vi "BMU诊断标定.vi"(5 "timeout":u32, 6 "Socket":dbl, 7 "通用配置?":bool, 8 "CAN端口":u16(ring), 9 "设备索引号":u16(ring), 10 "CAN卡类型":u32(ring)=21, 11 "从板号":u8=1) -> (3 "成功?":bool)   [LabVIEW 2013] (continued)
                              n874 = local write "正级继电器 8"(w1437) -> ()
                            }
                            frame 85, 170 {
                              n875 = local write "继电器超时处理"(TRUE ("继电器超时处理")) -> ()
                            }
                          }
                        }
                        frame 2 {
                          n876 = Index Array(array=w1453) -> (element #1=w1452:u8, element #2=w1451:u8, element #3=w1450:u8)  [unwired: 3 in]
                          n877 = Join Numbers(hi=w1451, lo=w1450) -> ((hi.lo)=w1449:u16)
                          n878 = case shown="2" w1452 {
                            tunnel: w1453 -> [_ _ _]
                            tunnel: w1449 -> [_ w1457 w1471]
                            tunnel: w1448 -> [_ w1456 _]
                            frame 0, Default {
                              n879 = local write "继电器超时处理"(FALSE ("继电器超时处理")) -> ()
                            }
                            frame 1 {
                              n880 = Equal To 0?(x=w1457) -> (x = 0?=w1455:bool)
                              n881 = case shown="假" w1455 {
                                tunnel: w1457 -> [w1463 _]
                                tunnel: [w1461 "DO控制操作成功!\nDO控制操作成功!\nDO控制操作成功!"] -> _
                                tunnel: w1456 -> [w1460 _]
                                frame False {
                                n882 = case shown="\"主板\", 默认" w1460 {
                                frame "主板", Default {
                                n883 = local read "DO1"() -> (w1466:bool)
                                n884 = Not(x=w1466) -> (.not. x?=w1465:bool)
                                n885 = local write "DO1"(w1465) -> ()
                                }
                                frame "从板" {
                                n886 = local read "DO1 2"() -> (w1468:bool)
                                n887 = Not(x=w1468) -> (.not. x?=w1467:bool)
                                n888 = local write "DO1 2"(w1467) -> ()
                                }
                                }
                                n889 = Number To Hexadecimal String(2:w1463) -> (0:w1462:string)  [unwired: 1 out]
                                n890 = Concatenate Strings("DO控制操作失败,0x" ("消息"), w1462) -> (w1461:string)
                                }
                                frame True {
                                }
                              }
                              n891 = case shown="\"从板\"" w1456 {
                                tunnel: w1455 -> [w1458 w1459]
                                frame "主板", Default {
                                n892 = local write "正级继电器 9"(w1458) -> ()
                                }
                                frame "从板" {
                                n893 = local write "正级继电器 11"(w1459) -> ()
                                }
                              }
                            }
                            frame 2 {
                              n894 = Equal To 0?(x=w1471) -> (x = 0?=w1470:bool)
                              n895 = case shown="假" w1470 {
                                tunnel: w1471 -> [w1476 _]
                                tunnel: [w1474 "DO控制操作成功!\nDO控制操作成功!\nDO控制操作成功!"] -> _
                                frame False {
                                n896 = Number To Hexadecimal String(2:w1476) -> (0:w1475:string)  [unwired: 1 out]
                                n897 = local read "DO2"() -> (w1473:bool)
                                n898 = Not(x=w1473) -> (.not. x?=w1472:bool)
                                n899 = Concatenate Strings("DO控制操作失败,0x" ("消息"), w1475) -> (w1474:string)
                                n900 = local write "DO2"(w1472) -> ()
                                }
                                frame True {
                                }
                              }
                              n901 = local write "正级继电器 10"(w1470) -> ()
                            }
                          }
                        }
                      }
                      n902 = local write "消除"(FALSE ("消除")) -> ()
                      n903 = global write "EV05全局变量1.vi" "流控帧 2"(FALSE ("流控帧 2")) -> ()
                      n904 = local write "控制1"(FALSE ("控制1")) -> ()
                      "继电器超时处理" <- TRUE ("控制1")
                    }
                  }
                }
                frame "高压板校正" {
                  n905 = local read "命令序号"() -> (w1483:u8)
                  n906 = call "多帧接收机制(EV05).vi"("can卡类型"=w1490, "设备索引号"=w1489, "CAN端口"=w1488, "VCI_Receive"=w1487, "命令"=w1485, "板号"=w1486, "命令序号"=w1483) -> ("错误信号"=w1479:bool, "错误代码"=w1492:i32, "输出数组"=w1484:u8[], "读错误代码"=w1482:u8[], "结束信号"=w1491:bool)  [unwired: 3 in, 5 out]
                  n907 = local read "控制1"() -> (w1480:bool)
                  n908 = And(x=w1480, y=w1491) -> (x .and. y?=w1481:bool)
                  n909 = case shown="真" w1481 {
                    tunnel: w1493 -> [_ w1497]
                    tunnel: w1492 -> [_ _]
                    tunnel: w1484 -> [_ w1495]
                    tunnel: w1483 -> [_ w1496]
                    tunnel: w1482 -> [_ w1498]
                    tunnel: w1479 -> [_ w1499]
                    frame False {
                    }
                    frame True {
                      n910 = case shown="假" w1499 {
                        tunnel: w1498 -> [_ w1709]
                        tunnel: w1497 -> [_ _]
                        tunnel: w1496 -> [w1504 _]
                        tunnel: w1495 -> [w1503 _]
                        frame False {
                          n911 = case shown="2" w1504 {
                            tunnel: w1503 -> [_ w1509 w1543 w1573 w1600 w1627 w1654 w1681]
                            frame 0, Default {
                            }
                            frame 1 {
                              n912 = for {
                                N: 10 -> [_]
                                tunnel: w1509 -> [w1526]
                                shift-right: [w1513] -> w1507
                                shift-left: string[] [] -> [w1515]
                                i -> [w1512]
                                w1520 = 8 ("索引")
                                w1524 = 2 ("y")
                                n913 = Multiply(x=w1512, y=w1524) -> (x*y=w1525:i32)
                                n914 = Array Subset(array=w1526, index=w1525, length=w1524) -> (w1523:u8[])
                                n915 = Index Array(array=w1523) -> (element #1=w1522:u8, element #2=w1521:u8)  [unwired: 2 in]
                                n916 = call "二进制解析-8.6.vi"("索引"=w1520, "数值"=w1522) -> ("低位子数组"=w1519:i32[])  [unwired: 1 in, 2 out]
                                n917 = call "二进制解析-8.6.vi"("索引"=w1520, "数值"=w1521) -> ("低位子数组"=w1518:i32[])  [unwired: 1 in, 2 out]
                                n918 = Insert Into Array(array=w1519, new element=w1518) -> (w1517:i32[])  [unwired: 1 in]
                                n919 = case shown="2" w1512 {
                                tunnel: [6 15 9 4 2 0 2] -> w1511
                                frame 0, Default {
                                }
                                frame 1 {
                                }
                                frame 2 {
                                }
                                frame 3..5 {
                                }
                                frame 8, 9 {
                                }
                                frame 7 {
                                }
                                frame 6 {
                                }
                                }
                                n920 = Reverse 1D Array(array=w1517) -> (reversed array=w1516:i32[])
                                n921 = for {
                                N: w1511 -> [_]
                                tunnel: w1516 -> [w1538] mode=indexing
                                tunnel: [w1534] -> w1514 mode=indexing
                                n922 = Equal To 0?(x=w1538) -> (x = 0?=w1537:bool)
                                n923 = Select(t="无", s=w1537, f="故障") -> (s? t:f=w1534:string)
                                }
                                n924 = Insert Into Array(array=w1515, new element=w1514) -> (w1513:string[])  [unwired: 1 in]
                              }
                              n925 = call "详细故障分解.vi"("名称"=string[] ["上电自检异常(CellV)", "通讯异常(CellV)", "不更新(CellV)", "未校准(CellV)", "保留", "采样线路断路(CellV)", "18b20上电自检异常(T) ", "18b20通讯异常(T)", "18b20传感器丢失(T)", "18b20传感器无号(T)", "18b20温度异常跳变(T)", "18b20信号线对电源短路(T)", "18b20信号线对地短路(T)", "18b20 CRC校验异常(T)", "NTC上电自检异常(T)", "NTC通讯异常(T)", "NTC传感器丢失(T)", "NTC温度异常跳变(T)", "NTC信号线断路(T)", "NTC信号线对电源短(T)", "NTC信号线对地短路(T)", "上电自检异常(Curr)", "参数异常(Curr)", "不更新(Curr)", "未校准(Curr)", "采样线断开(Curr)", "电流零漂异常(Curr)", "传感器反接(Curr)", "读取实时电流故障(Curr)", "平均电流故障(Curr)", "自检异常(iso)", "前端检测电阻损坏(iso)", "不更新(iso)", "未校准(iso)", "上电自检异常(Sumv_in)", "通讯异常(Sumv_in)", "不更新(Sumv_in)", "未校准(Sumv_in)", "上电自检异常(Sumv_out)", "通讯异常(Sumv_out)", "不更新(Sumv_out)", "未校准(Sumv_out)", "系统时钟自检异常(Clock)", "系统时钟未校准(Clock)", "充电均衡模块不能开启", "充电均衡模块不能关闭", "放电均衡模块不能开启", "放电均衡模块不能关闭"], "故障输入口"=w1507) -> ("输出数组"=w1505:string[][])  [unwired: 1 in, 2 out]
                              n926 = local write "电池故障"(w1505) -> ()
                            }
                            frame 2 {
                              n927 = for {
                                N: 5 -> [_]
                                tunnel: w1543 -> [w1560]
                                shift-right: [w1547] -> w1541
                                shift-left: string[] [] -> [w1549]
                                i -> [w1545]
                                w1554 = 8 ("索引")
                                w1558 = 2 ("y")
                                n928 = Multiply(x=w1545, y=w1558) -> (x*y=w1559:i32)
                                n929 = Array Subset(array=w1560, index=w1559, length=w1558) -> (w1557:u8[])
                                n930 = Index Array(array=w1557) -> (element #1=w1556:u8, element #2=w1555:u8)  [unwired: 2 in]
                                n931 = call "二进制解析-8.6.vi"("索引"=w1554, "数值"=w1556) -> ("低位子数组"=w1553:i32[])  [unwired: 1 in, 2 out]
                                n932 = call "二进制解析-8.6.vi"("索引"=w1554, "数值"=w1555) -> ("低位子数组"=w1552:i32[])  [unwired: 1 in, 2 out]
                                n933 = Insert Into Array(array=w1553, new element=w1552) -> (w1551:i32[])  [unwired: 1 in]
                                n934 = case shown="2" w1545 {
                                tunnel: [4 6 5] -> w1546
                                frame 0, Default {
                                }
                                frame 2 {
                                }
                                frame 4 {
                                }
                                }
                                n935 = Reverse 1D Array(array=w1551) -> (reversed array=w1550:i32[])
                                n936 = for {
                                N: w1546 -> [_]
                                tunnel: w1550 -> [w1568] mode=indexing
                                tunnel: [w1564] -> w1548 mode=indexing
                                n937 = Equal To 0?(x=w1568) -> (x = 0?=w1567:bool)
                                n938 = Select(t="无", s=w1567, f="故障") -> (s? t:f=w1564:string)
                                }
                                n939 = Insert Into Array(array=w1549, new element=w1548) -> (w1547:string[])  [unwired: 1 in]
                              }
                              n940 = call "详细故障分解.vi"("名称"=string[] ["自检异常(ee_cpu)", "存储空间满(ee_cpu)", "数据写入失败(ee_cpu)", "数据读取异常(ee_cpu)", "自检异常(ee_ext)", "存储空间满(ee_ext)", "数据写入失败(ee_ext)", "数据读取异常(ee_ext)", "自检异常(flash_ext)", "故障数据存储空间满(flash_ext)", "历史数据存储空间满(flash_ext)", "数据写入失败(flash_ext)", "数据读取失败(flash_ext)", "数据校验异常(flash_ext)", "自检异常(flash_cpu)", "存储空间满(flash_cpu)", "数据写入失败(flash_cpu)", "数据读取异常(flash_cpu)", "应用程序异常(cpu)", "应用程序下载异常(cpu)", "AD模块异常(cpu)", "RAM异常(cpu)", "CPU异常下电(cpu)"], "故障输入口"=w1541) -> ("输出数组"=w1539:string[][])  [unwired: 1 in, 2 out]
                              n941 = local write "电池故障"(w1539) -> ()
                            }
                            frame 3 {
                              n942 = for {
                                N: 5 -> [_]
                                tunnel: w1573 -> [w1590]
                                shift-right: [w1577] -> w1571
                                shift-left: string[] [] -> [w1579]
                                i -> [w1576]
                                w1584 = 8 ("索引")
                                w1588 = 2 ("y")
                                n943 = Multiply(x=w1576, y=w1588) -> (x*y=w1589:i32)
                                n944 = Array Subset(array=w1590, index=w1589, length=w1588) -> (w1587:u8[])
                                n945 = Index Array(array=w1587) -> (element #1=w1586:u8, element #2=w1585:u8)  [unwired: 2 in]
                                n946 = call "二进制解析-8.6.vi"("索引"=w1584, "数值"=w1586) -> ("低位子数组"=w1583:i32[])  [unwired: 1 in, 2 out]
                                n947 = call "二进制解析-8.6.vi"("索引"=w1584, "数值"=w1585) -> ("低位子数组"=w1582:i32[])  [unwired: 1 in, 2 out]
                                n948 = Insert Into Array(array=w1583, new element=w1582) -> (w1581:i32[])  [unwired: 1 in]
                                n949 = Reverse 1D Array(array=w1581) -> (reversed array=w1580:i32[])
                                n950 = for {
                                N: 6 -> [_]
                                tunnel: w1580 -> [w1595] mode=indexing
                                tunnel: [w1591] -> w1578 mode=indexing
                                n951 = Equal To 0?(x=w1595) -> (x = 0?=w1594:bool)
                                n952 = Select(t="无", s=w1594, f="故障") -> (s? t:f=w1591:string)
                                }
                                n953 = Insert Into Array(array=w1579, new element=w1578) -> (w1577:string[])  [unwired: 1 in]
                              }
                              n954 = call "详细故障分解.vi"("名称"=string[] ["初始化失败(CAN4)", "发送异常(CAN4)", "接收异常(CAN4)", "总线超时(CAN4)", "BUSOFF(CAN4)", "帧格式(CAN4)", "初始化异常(CAN0)", "发送异常(CAN0)", "接收异常(CAN0)", "总线超时(CAN0)", "BUSOFF(CAN0)", "帧格式(CAN0)", "初始化异常(CAN1)", "发送异常(CAN1)", "接收异常(CAN1)", "总线超时(CAN1)", "BUSOFF(CAN1)", "帧格式(CAN1)", "初始化失败(CAN2)", "发送异常(CAN2)", "接收异常(CAN2)", "总线超时(CAN2)", "BUSOFF(CAN2)", "帧格式(CAN2)", "初始化失败(CAN3)", "发送异常(CAN3)", "接收异常(CAN3)", "总线超时(CAN3)", "BUSOFF(CAN3)", "帧格式(CAN3)"], "故障输入口"=w1571) -> ("输出数组"=w1569:string[][])  [unwired: 1 in, 2 out]
                              n955 = local write "电池故障"(w1569) -> ()
                            }
                            frame 4 {
                              n956 = for {
                                N: 1 -> [_]
                                tunnel: w1600 -> [w1617]
                                shift-right: [w1604] -> w1598
                                shift-left: string[] [] -> [w1606]
                                i -> [w1603]
                                w1611 = 8 ("索引")
                                w1615 = 2 ("y")
                                n957 = Multiply(x=w1603, y=w1615) -> (x*y=w1616:i32)
                                n958 = Array Subset(array=w1617, index=w1616, length=w1615) -> (w1614:u8[])
                                n959 = Index Array(array=w1614) -> (element #1=w1613:u8, element #2=w1612:u8)  [unwired: 2 in]
                                n960 = call "二进制解析-8.6.vi"("索引"=w1611, "数值"=w1613) -> ("低位子数组"=w1610:i32[])  [unwired: 1 in, 2 out]
                                n961 = call "二进制解析-8.6.vi"("索引"=w1611, "数值"=w1612) -> ("低位子数组"=w1609:i32[])  [unwired: 1 in, 2 out]
                                n962 = Insert Into Array(array=w1610, new element=w1609) -> (w1608:i32[])  [unwired: 1 in]
                                n963 = Reverse 1D Array(array=w1608) -> (reversed array=w1607:i32[])
                                n964 = for {
                                N: 4 -> [_]
                                tunnel: w1607 -> [w1622] mode=indexing
                                tunnel: [w1618] -> w1605 mode=indexing
                                n965 = Equal To 0?(x=w1622) -> (x = 0?=w1621:bool)
                                n966 = Select(t="无", s=w1621, f="故障") -> (s? t:f=w1618:string)
                                }
                                n967 = Insert Into Array(array=w1606, new element=w1605) -> (w1604:string[])  [unwired: 1 in]
                              }
                              n968 = call "详细故障分解.vi"("名称"=string[] ["通讯协议版本不一致(soft)", "系统不同步(soft)", "软件版本不一致(soft)", "同硬件平台不兼容(soft)"], "故障输入口"=w1598) -> ("输出数组"=w1596:string[][])  [unwired: 1 in, 2 out]
                              n969 = local write "电池故障"(w1596) -> ()
                            }
                            frame 5 {
                              n970 = for {
                                N: 2 -> [_]
                                tunnel: w1627 -> [w1644]
                                shift-right: [w1631] -> w1625
                                shift-left: string[] [] -> [w1633]
                                i -> [w1630]
                                w1638 = 8 ("索引")
                                w1642 = 2 ("y")
                                n971 = Multiply(x=w1630, y=w1642) -> (x*y=w1643:i32)
                                n972 = Array Subset(array=w1644, index=w1643, length=w1642) -> (w1641:u8[])
                                n973 = Index Array(array=w1641) -> (element #1=w1640:u8, element #2=w1639:u8)  [unwired: 2 in]
                                n974 = call "二进制解析-8.6.vi"("索引"=w1638, "数值"=w1640) -> ("低位子数组"=w1637:i32[])  [unwired: 1 in, 2 out]
                                n975 = call "二进制解析-8.6.vi"("索引"=w1638, "数值"=w1639) -> ("低位子数组"=w1636:i32[])  [unwired: 1 in, 2 out]
                                n976 = Insert Into Array(array=w1637, new element=w1636) -> (w1635:i32[])  [unwired: 1 in]
                                n977 = Reverse 1D Array(array=w1635) -> (reversed array=w1634:i32[])
                                n978 = for {
                                N: 4 -> [_]
                                tunnel: w1634 -> [w1649] mode=indexing
                                tunnel: [w1645] -> w1632 mode=indexing
                                n979 = Equal To 0?(x=w1649) -> (x = 0?=w1648:bool)
                                n980 = Select(t="无", s=w1648, f="故障") -> (s? t:f=w1645:string)
                                }
                                n981 = Insert Into Array(array=w1633, new element=w1632) -> (w1631:string[])  [unwired: 1 in]
                              }
                              n982 = call "详细故障分解.vi"("名称"=string[] ["初始化失败(RS232)", "发送异常(RS232)", "接收异常(RS232)", "总线超时(RS232)", "初始化失败(RS485)", "发送异常(RS485)", "接收异常(RS485)", "总线超时(RS485)"], "故障输入口"=w1625) -> ("输出数组"=w1623:string[][])  [unwired: 1 in, 2 out]
                              n983 = local write "电池故障"(w1623) -> ()
                            }
                            frame 6 {
                              n984 = for {
                                N: 2 -> [_]
                                tunnel: w1654 -> [w1671]
                                shift-right: [w1658] -> w1652
                                shift-left: string[] [] -> [w1660]
                                i -> [w1657]
                                w1665 = 8 ("索引")
                                w1669 = 2 ("y")
                                n985 = Multiply(x=w1657, y=w1669) -> (x*y=w1670:i32)
                                n986 = Array Subset(array=w1671, index=w1670, length=w1669) -> (w1668:u8[])
                                n987 = Index Array(array=w1668) -> (element #1=w1667:u8, element #2=w1666:u8)  [unwired: 2 in]
                                n988 = call "二进制解析-8.6.vi"("索引"=w1665, "数值"=w1667) -> ("低位子数组"=w1664:i32[])  [unwired: 1 in, 2 out]
                                n989 = call "二进制解析-8.6.vi"("索引"=w1665, "数值"=w1666) -> ("低位子数组"=w1663:i32[])  [unwired: 1 in, 2 out]
                                n990 = Insert Into Array(array=w1664, new element=w1663) -> (w1662:i32[])  [unwired: 1 in]
                                n991 = Reverse 1D Array(array=w1662) -> (reversed array=w1661:i32[])
                                n992 = for {
                                N: 16 -> [_]
                                tunnel: w1661 -> [w1676] mode=indexing
                                tunnel: [w1672] -> w1659 mode=indexing
                                n993 = Equal To 0?(x=w1676) -> (x = 0?=w1675:bool)
                                n994 = Select(t="无", s=w1675, f="故障") -> (s? t:f=w1672:string)
                                }
                                n995 = Insert Into Array(array=w1660, new element=w1659) -> (w1658:string[])  [unwired: 1 in]
                              }
                              n996 = call "详细故障分解.vi"("名称"=string[] ["DI1对地短", "DI1对电源短", "DI2对地短", "DI2对电源短", "DI3对地短", "DI3对电源短", "DI4对地短", "DI4对电源短", "DI5对地短", "DI5对电源短", "DI6对地短", "DI6对电源短", "DI7对地短", "DI7对电源短", "DI8对地短", "DI8对电源短", "DO1对地短", "DO1对电源短", "DO2对地短", "DO2对电源短", "DO3对地短", "DO3对电源短", "DO4对地短", "DO4对电源短", "DO5对地短", "DO5对电源短", "DO6对地短", "DO6对电源短", "DO7对地短", "DO7对电源短", "DO8对地短", "DO8对电源短"], "故障输入口"=w1652) -> ("输出数组"=w1650:string[][])  [unwired: 1 in, 2 out]
                              n997 = local write "电池故障"(w1650) -> ()
                            }
                            frame 7 {
                              n998 = for {
                                N: 2 -> [_]
                                tunnel: w1681 -> [w1698]
                                shift-right: [w1685] -> w1679
                                shift-left: string[] [] -> [w1687]
                                i -> [w1683]
                                w1692 = 8 ("索引")
                                w1696 = 2 ("y")
                                n999 = Multiply(x=w1683, y=w1696) -> (x*y=w1697:i32)
                                n1000 = Array Subset(array=w1698, index=w1697, length=w1696) -> (w1695:u8[])
                                n1001 = Index Array(array=w1695) -> (element #1=w1694:u8, element #2=w1693:u8)  [unwired: 2 in]
                                n1002 = call "二进制解析-8.6.vi"("索引"=w1692, "数值"=w1694) -> ("低位子数组"=w1691:i32[])  [unwired: 1 in, 2 out]
                                n1003 = call "二进制解析-8.6.vi"("索引"=w1692, "数值"=w1693) -> ("低位子数组"=w1690:i32[])  [unwired: 1 in, 2 out]
                                n1004 = Insert Into Array(array=w1691, new element=w1690) -> (w1689:i32[])  [unwired: 1 in]
                                n1005 = case shown="1" w1683 {
                                tunnel: [4 6] -> w1684
                                frame 0, Default {
                                }
                                frame 1 {
                                }
                                }
                                n1006 = Reverse 1D Array(array=w1689) -> (reversed array=w1688:i32[])
                                n1007 = for {
                                N: w1684 -> [_]
                                tunnel: w1688 -> [w1705] mode=indexing
                                tunnel: [w1701] -> w1686 mode=indexing
                                n1008 = Equal To 0?(x=w1705) -> (x = 0?=w1704:bool)
                                n1009 = Select(t="无", s=w1704, f="故障") -> (s? t:f=w1701:string)
                                }
                                n1010 = Insert Into Array(array=w1687, new element=w1686) -> (w1685:string[])  [unwired: 1 in]
                              }
                              n1011 = call "详细故障分解.vi"("名称"=string[] ["超时(pre-chg)", "后端开路(pre-chg)", "后端短路(pre-chg)", "预充电回路断开(pre-chg)", "正级继电器驱动故障(relay_driver)", "负级继电器驱动故障(relay_driver)", "预充电继电器驱动故障(relay_driver)", "充电继电器驱动故障(relay_driver)", "风机继电器驱动故障(relay_driver)", "加热继电器驱动故障(relay_driver)"], "故障输入口"=w1679) -> ("输出数组"=w1677:string[][])  [unwired: 1 in, 2 out]
                              n1012 = local write "电池故障"(w1677) -> ()
                            }
                          }
                        }
                        frame True {
                          n1013 = Index Array(array=w1709, index #1=0 ("索引"), index #2=1 ("索引")) -> (element #1=w1712:u8, element #2=w1713:u8)
                          n1014 = Join Numbers(hi=w1712, lo=w1713) -> ((hi.lo)=w1711:u16)
                          n1015 = Number To Hexadecimal String(2:w1711) -> (0:w1710:string)  [unwired: 1 out]
                          n1016 = Concatenate Strings("读取错误，代码： " ("字符串"), "0x" ("字符串"), w1710) -> (w1708:string)
                          n1017 = One Button Dialog(message=w1708, button name ("OK")="是" ("按钮名称（“确定”）")) -> ()  [unwired: 1 out]
                        }
                      }
                      n1018 = local write "消除"(FALSE ("消除")) -> ()
                      n1019 = global write "EV05全局变量1.vi" "流控帧 2"(FALSE ("流控帧 2")) -> ()
                      n1020 = local write "控制1"(FALSE ("控制1")) -> ()
                      n1021 = global write "EV05全局变量1.vi" "写入超时"(TRUE ("写入超时")) -> ()
                    }
                  }
                }
              }
            }
          }
        }
      }
      frame Error {
      }
    }
  }
  n1022 = disable-structure shown="启用" {
    disable-tunnel: w79 -> [w1725 _]
    disable-tunnel: w50 -> [w1724 _]
    disable-tunnel: w36 -> [w1719 _]
    disable-tunnel: w41 -> [w1718 _]
    disable-tunnel: w4 -> [w1717 _]
    frame Enabled {
      n1023 = while {
        tunnel: w1725 -> [w1734]
        tunnel: w1724 -> [w1733]
        tunnel: [w1732] -> w1723
        tunnel: [w1731] -> w1722
        tunnel: w1719 -> [_]
        tunnel: w1718 -> [_]
        tunnel: w1717 -> [w1729]
        stop <- w1726 stop-if-true
        n1024 = event shown="[0] 超时" {
          selector: _ -> [_ _ _ _ _ _ _ _ _ _ _ _ _ _ _ _ _ _ _ _ _ _ _ _ _ _ _ _ _ _ _ _ _ _ _ _ _ _ _ _ _ _ _ _ _ _ _ _ _ _ _ _ _]
          dyn-events: _ -> [_ _ _ _ _ _ _ _ _ _ _ _ _ _ _ _ _ _ _ _ _ _ _ _ _ _ _ _ _ _ _ _ _ _ _ _ _ _ _ _ _ _ _ _ _ _ _ _ _ _ _ _ _]
          timeout: 200 -> [_ _ _ _ _ _ _ _ _ _ _ _ _ _ _ _ _ _ _ _ _ _ _ _ _ _ _ _ _ _ _ _ _ _ _ _ _ _ _ _ _ _ _ _ _ _ _ _ _ _ _ _ _]
          tunnel: [w1738 w1744 w1784 _ _ _ _ _ _ _ _ _ _ _ _ _ _ _ _ _ _ _ _ _ _ _ _ _ _ _ _ _ _ _ _ _ _ _ _ _ _ _ _ _ _ _ _ _ _ _ _ _ _] -> w1727
          tunnel: w1734 -> [w1743 w1747 w1783 _ w1824 w1835 w1846 w1857 w1868 w1879 w1890 w1901 w1912 w1923 w1934 w1945 w1961 w2484 w2896 w2921 w2949 w3052 w3125 w3138 w3148 w3194 _ _ w3244 w3311 w3378 w3445 w3512 w3579 w3646 w3714 w3782 w3849 w3916 w3986 w3997 w4036 w4076 w4116 w4156 w4194 w4254 w4289 w4325 w4358 w4428 w4461 w4494]
          tunnel: w1733 -> [w1742 w1746 w1782 _ w1823 w1834 w1845 w1856 w1867 w1878 w1889 w1900 w1911 w1922 w1933 w1944 w1960 w2483 w2895 w2920 w2948 w3051 w3123 w3136 w3147 w3193 _ _ w3243 w3310 w3377 w3444 w3511 w3578 w3645 w3713 w3781 w3848 w3915 w3984 w3996 w4035 w4075 w4115 w4155 w4193 w4253 w4288 w4324 w4357 w4427 w4460 w4493]
          tunnel: [w1743 w1747 w1783 _ w1824 w1835 w1846 w1857 w1868 w1879 w1890 w1901 w1912 w1923 w1934 w1945 w1961 w2484 w2896 w2921 w2949 w3052 w3124 w3137 w3148 w3194 _ _ w3244 w3311 w3378 w3445 w3512 w3579 w3646 w3714 w3782 w3849 w3916 w3985 w3995 w4034 w4074 w4114 w4154 w4194 w4252 w4287 w4323 w4356 w4426 w4459 w4492] -> w1732
          tunnel: [w1742 w1746 w1782 _ w1823 w1834 w1845 w1856 w1867 w1878 w1889 w1900 w1911 w1922 w1933 w1944 w1960 w2483 w2895 w2920 w2948 w3051 w3122 w3135 w3147 w3193 _ _ w3243 w3310 w3377 w3444 w3511 w3578 w3645 w3713 w3781 w3848 w3915 w3983 w3994 w4033 w4073 w4113 w4153 w4193 w4251 w4286 w4322 w4355 w4425 w4458 w4491] -> w1731
          tunnel: [_ _ _ _ _ _ _ _ _ _ _ _ _ _ _ _ _ _ _ _ _ _ _ _ _ _ _ _ _ _ _ _ _ _ _ _ _ _ _ _ w3994 w4033 w4073 w4113 w4153 _ w4251 w4286 w4322 w4355 w4425 w4458 w4491] -> _
          tunnel: w1729 -> [w1740 _ _ _ _ _ _ _ _ _ _ _ _ _ _ _ _ _ _ _ _ _ _ _ _ _ _ _ _ _ _ _ _ _ _ _ _ _ _ _ _ _ _ _ _ _ _ _ _ _ _ _ _]
          event Timeout {
            n1025 = event-data() -> ()  [unwired: 3 out]
            n1026 = Tick Count (ms)() -> (millisecond timer value=w1741:u32)
            n1027 = Subtract(x=w1741, y=w1740) -> (x-y=w1737:u32)
            n1028 = Divide(x=w1737, y=u32 1000) -> (x/y=→"x/y":dbl)
            n1029 = Greater Or Equal?(x=w1737, y="timeout") -> (x >= y?=w1738:bool)
            "timeout" <- w1738
          }
          event "停止": Value Change {
            n1030 = event-data() -> ("NewVal"=w1745:bool)  [unwired: 5 out]
            n1031 = stacked-sequence {
              tunnel: w1745 -> [w1764 _]
              tunnel: [w1764 _] -> w1744
              frame #0 {
                n1032 = global read "配置文件全局.vi" "诊断标定读取地址"() -> (w1748:path)
                n1033 = call <vilib>:"Application Directory.vi"() -> ("Application Directory"=w1758:path)
                n1034 = property class="VI"("FP.State"=T26."Hidden" ("前面板窗口:状态")) -> (reference out=w1760:refnum<vi>, error out=w1759:errorcluster)  [unwired: 2 in]
                n1035 = Build Path(base path=w1758, name or relative path="config.ini" ("名称或相对路径")) -> (appended path=w1756:path)
                n1036 = call <vilib>:"Open Config Data.vi"("configuration file path"=w1756) -> ("error out"=w1753:errorcluster, "refnum"=w1755:T19)  [unwired: 8 in, 1 out]
                n1037 = local write "停止"(TRUE ("停止")) -> ()
                n1038 = property class="VI"(reference=w1760, error in=w1759, "Front Panel.Open"=FALSE ("前面板窗口:打开")) -> ()  [unwired: 2 out]
                n1039 = call-poly <vilib>:"Write Key.vi"("section"="总信息", "error in (no error)"=w1753, "value"=w1748, "key"="诊断标定读取地址" ("section"), "refnum"=w1755) -> ("error out"=w1752:errorcluster, "refnum out"=w1751:T19)  [unwired: 4 in, 1 out]
                n1040 = call <vilib>:"Close Config Data.vi"("error in (no error)"=w1752, "refnum"=w1751) -> ("error out"=w1750:errorcluster)  [unwired: 8 in, 1 out]
                n1041 = call <vilib>:"Clear Errors.vi"("error in (no error)"=w1750) -> ()  [unwired: 6 in, 1 out]
              }
              frame #1 {
                n1042 = disable-structure shown="禁用" {
                  frame Disabled {
                    n1043 = local read "设备索引号"() -> (w1770:u16)
                    n1044 = local read "CAN卡类型"() -> (w1771:u32)
                    n1045 = local read "CAN端口"() -> (w1769:u16)
                    n1046 = Build Array(7) -> (w1766:i32[])
                    n1047 = call "transmit-8.6.vi"("can卡类型"=w1771, "设备索引号"=w1770, "CAN端口"=w1769, "ID"=418398080, "SendType"=u8 0, "Data"=w1766) -> ()  [unwired: 3 in, 11 out]
                  }
                  frame Enabled {
                    w1778 = u8 0 items=["Normal", "Listen Only"] ("工作方式")
                    w1777 = u8 1 items=["Dual Filter", "Single Filter"] ("滤波方式")
                    n1048 = local read "设备索引号"() -> (w1773:u16)
                    n1049 = local read "CAN卡类型"() -> (w1772:u32)
                    n1050 = local read "CAN端口"() -> (w1774:u16)
                    n1051 = call "CAN_Init-8.6.vi"("CAN卡类型"=w1772, "设备索引号"=w1773, "CAN端口"=w1774, "操作类型"=enum16{"初始化CAN", "关闭CAN"}."初始化CAN", "滤波方式"=w1777, "Accept Code"=u32 0, "簇"=T23 {"打开CAN"=FALSE, "初始化CAN"=TRUE, "开始CAN"=TRUE, "重启"=FALSE, "关闭CAN"=FALSE}, "Mask Code"=u32 4294967295 ("Accept Code"), "工作方式"=w1778, "是否滤波"=FALSE) -> ()  [unwired: 4 in, 6 out]
                  }
                }
              }
            }
          }
          event Panel Close? {
            n1052 = event-data() -> ()  [unwired: 5 out]
            n1053 = stacked-sequence {
              tunnel: [w1797 _] -> w1784
              frame #0 {
                w1797 = TRUE ("前面板窗口:打开")
                n1054 = global read "配置文件全局.vi" "诊断标定读取地址"() -> (w1786:path)
                n1055 = call <vilib>:"Application Directory.vi"() -> ("Application Directory"=w1796:path)
                n1056 = property class="VI"("FP.State"=T26."Hidden" ("前面板窗口:状态")) -> (reference out=w1799:refnum<vi>, error out=w1798:errorcluster)  [unwired: 2 in]
                n1057 = Build Path(base path=w1796, name or relative path="config.ini" ("名称或相对路径")) -> (appended path=w1794:path)
                n1058 = call <vilib>:"Open Config Data.vi"("configuration file path"=w1794) -> ("error out"=w1791:errorcluster, "refnum"=w1793:T19)  [unwired: 8 in, 1 out]
                n1059 = property class="VI"(reference=w1799, error in=w1798, "Front Panel.Open"=FALSE ("前面板窗口:打开")) -> ()  [unwired: 2 out]
                n1060 = call-poly <vilib>:"Write Key.vi"("section"="总信息", "error in (no error)"=w1791, "value"=w1786, "key"="诊断标定读取地址" ("section"), "refnum"=w1793) -> ("error out"=w1790:errorcluster, "refnum out"=w1789:T19)  [unwired: 4 in, 1 out]
                n1061 = call <vilib>:"Close Config Data.vi"("error in (no error)"=w1790, "refnum"=w1789) -> ("error out"=w1788:errorcluster)  [unwired: 8 in, 1 out]
                n1062 = call <vilib>:"Clear Errors.vi"("error in (no error)"=w1788) -> ()  [unwired: 6 in, 1 out]
                n1063 = local write "强制终止读写标记"(TRUE ("强制终止读写标记")) -> ()
                n1064 = local write "停止"(w1797) -> ()
              }
              frame #1 {
                w1805 = u8 0 items=["Normal", "Listen Only"] ("工作方式")
                w1806 = u8 1 items=["Dual Filter", "Single Filter"] ("滤波方式")
                n1065 = local read "设备索引号"() -> (w1810:u16)
                n1066 = local read "CAN卡类型"() -> (w1811:u32)
                n1067 = local read "CAN端口"() -> (w1809:u16)
                n1068 = call "CAN_Init-8.6.vi"("CAN卡类型"=w1811, "设备索引号"=w1810, "CAN端口"=w1809, "操作类型"=enum16{"初始化CAN", "关闭CAN"}."初始化CAN", "滤波方式"=w1806, "Accept Code"=u32 0, "簇"=T23 {"打开CAN"=FALSE, "初始化CAN"=TRUE, "开始CAN"=TRUE, "重启"=FALSE, "关闭CAN"=FALSE}, "Mask Code"=u32 4294967295 ("Accept Code"), "工作方式"=w1805, "是否滤波"=FALSE) -> ()  [unwired: 4 in, 6 out]
              }
            }
            n1069 = event-data("Discard?"=w1784) -> ()  [unwired: 1 in, 1 out]
          }
          event "终止读写按钮": Value Change {
            n1070 = event-data() -> ("NewVal"=w1812:bool)  [unwired: 6 out]
            n1071 = case shown="真" w1812 {
              frame False {
              }
              frame True {
                n1072 = local write "强制终止读写标记"(TRUE ("强制终止读写标记")) -> ()
              }
            }
          }
          event "1": Value Change {
            w1821 = FALSE ("1")
            n1073 = event-data() -> ()  [unwired: 7 out]
            n1074 = local write "主板2"(T8."项目信息" ("主从板")) -> ()
            n1075 = Not(x=w1821) -> (.not. x?=w1820:bool)
            n1076 = local write "1"(w1820) -> ()
            n1077 = local write "1 2"(w1821) -> ()
            n1078 = local write "1 3"(w1821) -> ()
            n1079 = local write "1 4"(w1821) -> ()
            n1080 = local write "1 5"(w1821) -> ()
            n1081 = local write "1 11"(w1821) -> ()
            n1082 = global read "功能码全局.vi" "主板监控2"() -> (w1819:bool[])
            n1083 = Index Array(array=w1819, index=6 ("索引")) -> (element=w1814:bool)
            n1084 = Select(t=0, s=w1814, f=1) -> (s? t:f=w1815:i32)
            n1085 = property on="项目信息" class="Tbl (严格)"("Disabled"=w1815) -> ()  [unwired: 2 in, 2 out]
            n1086 = property on="电池实际容量(A)" class="DigNum (严格)"("Disabled"=w1815) -> ()  [unwired: 2 in, 2 out]
            n1087 = property on="使用者" class="DigNum (严格)"("Disabled"=w1815) -> ()  [unwired: 2 in, 2 out]
            n1088 = property on="SOH(%)" class="DigNum (严格)"("Disabled"=w1815) -> ()  [unwired: 2 in, 2 out]
            n1089 = property on="电池额定容量(A)" class="DigNum (严格)"("Disabled"=w1815) -> ()  [unwired: 2 in, 2 out]
            n1090 = property on="SOC(%)" class="DigNum (严格)"("Disabled"=w1815) -> ()  [unwired: 2 in, 2 out]
            n1091 = property on="项目信息2" class="Clust (严格)"("DisabledEnum"=w1815) -> ()  [unwired: 2 in, 2 out]
            n1092 = property on="系统时钟" class="Str"("Disabled"=w1815) -> ()  [unwired: 2 in, 2 out]
            n1093 = property on="配置文件版本" class="Str"("Disabled"=w1815) -> ()  [unwired: 2 in, 2 out]
            n1094 = property on="车架(牌)号" class="Str"("Disabled"=w1815) -> ()  [unwired: 2 in, 2 out]
            n1095 = property on="产品编号" class="Str"("Disabled"=w1815) -> ()  [unwired: 2 in, 2 out]
          }
          event "1 2": Value Change {
            w1832 = FALSE ("1")
            n1096 = event-data() -> ()  [unwired: 7 out]
            n1097 = local write "主板2"(T8."一级故障阀值" ("主从板")) -> ()
            n1098 = Not(x=w1832) -> (.not. x?=w1831:bool)
            n1099 = local write "1"(w1832) -> ()
            n1100 = local write "1 2"(w1831) -> ()
            n1101 = local write "1 3"(w1832) -> ()
            n1102 = local write "1 4"(w1832) -> ()
            n1103 = local write "1 5"(w1832) -> ()
            n1104 = local write "1 11"(w1832) -> ()
            n1105 = global read "功能码全局.vi" "主板监控2"() -> (w1830:bool[])
            n1106 = Index Array(array=w1830, index=6 ("索引")) -> (element=w1825:bool)
            n1107 = Select(t=0, s=w1825, f=1) -> (s? t:f=w1828:i32)
            n1108 = property on="一级故障" class="Clust (严格)"("DisabledEnum"=w1828) -> ()  [unwired: 2 in, 2 out]
          }
          event "1 3": Value Change {
            w1843 = FALSE ("1")
            n1109 = event-data() -> ()  [unwired: 7 out]
            n1110 = local write "主板2"(T8."二级故障阀值" ("主从板")) -> ()
            n1111 = Not(x=w1843) -> (.not. x?=w1842:bool)
            n1112 = local write "1"(w1843) -> ()
            n1113 = local write "1 2"(w1843) -> ()
            n1114 = local write "1 3"(w1842) -> ()
            n1115 = local write "1 4"(w1843) -> ()
            n1116 = local write "1 5"(w1843) -> ()
            n1117 = local write "1 11"(w1843) -> ()
            n1118 = global read "功能码全局.vi" "主板监控2"() -> (w1841:bool[])
            n1119 = Index Array(array=w1841, index=6 ("索引")) -> (element=w1837:bool)
            n1120 = Select(t=0, s=w1837, f=1) -> (s? t:f=w1836:i32)
            n1121 = property on="一级故障 2" class="Clust (严格)"("DisabledEnum"=w1836) -> ()  [unwired: 2 in, 2 out]
          }
          event "1 4": Value Change {
            w1854 = FALSE ("1")
            n1122 = event-data() -> ()  [unwired: 7 out]
            n1123 = local write "主板2"(T8."三级故障阀值" ("主从板")) -> ()
            n1124 = Not(x=w1854) -> (.not. x?=w1853:bool)
            n1125 = local write "1"(w1854) -> ()
            n1126 = local write "1 2"(w1854) -> ()
            n1127 = local write "1 3"(w1854) -> ()
            n1128 = local write "1 4"(w1853) -> ()
            n1129 = local write "1 5"(w1854) -> ()
            n1130 = local write "1 11"(w1854) -> ()
            n1131 = global read "功能码全局.vi" "主板监控2"() -> (w1852:bool[])
            n1132 = Index Array(array=w1852, index=6 ("索引")) -> (element=w1847:bool)
            n1133 = Select(t=0, s=w1847, f=1) -> (s? t:f=w1850:i32)
            n1134 = property on="一级故障 3" class="Clust (严格)"("DisabledEnum"=w1850) -> ()  [unwired: 2 in, 2 out]
          }
          event "1 5": Value Change {
            w1865 = FALSE ("1")
            n1135 = event-data() -> ()  [unwired: 7 out]
            n1136 = local write "主板2"(T8."控制参数" ("主从板")) -> ()
            n1137 = Not(x=w1865) -> (.not. x?=w1864:bool)
            n1138 = local write "1"(w1865) -> ()
            n1139 = local write "1 2"(w1865) -> ()
            n1140 = local write "1 3"(w1865) -> ()
            n1141 = local write "1 4"(w1865) -> ()
            n1142 = local write "1 5"(w1864) -> ()
            n1143 = local write "1 11"(w1865) -> ()
            n1144 = global read "功能码全局.vi" "主板监控2"() -> (w1861:bool[])
            n1145 = Index Array(array=w1861, index=6 ("索引")) -> (element=w1859:bool)
            n1146 = Select(t=0, s=w1859, f=1) -> (s? t:f=w1858:i32)
            n1147 = property on="风机开启温度" class="DigNum (严格)"("Disabled"=w1858) -> ()  [unwired: 2 in, 2 out]
            n1148 = property on="风机关闭温度" class="DigNum (严格)"("Disabled"=w1858) -> ()  [unwired: 2 in, 2 out]
            n1149 = property on="加热开启温度" class="DigNum (严格)"("Disabled"=w1858) -> ()  [unwired: 2 in, 2 out]
            n1150 = property on="加热关闭温度" class="DigNum (严格)"("Disabled"=w1858) -> ()  [unwired: 2 in, 2 out]
            n1151 = property on="风机开启温差" class="DigNum (严格)"("Disabled"=w1858) -> ()  [unwired: 2 in, 2 out]
            n1152 = property on="风机关闭温差" class="DigNum (严格)"("Disabled"=w1858) -> ()  [unwired: 2 in, 2 out]
            n1153 = property on="加热控制参数" class="Clust (严格)"("DisabledEnum"=w1858) -> ()  [unwired: 2 in, 2 out]
            n1154 = property on="最大允许总电压" class="DigNum (严格)"("Disabled"=w1858) -> ()  [unwired: 2 in, 2 out]
            n1155 = property on="最大允许充电温度" class="DigNum (严格)"("Disabled"=w1858) -> ()  [unwired: 2 in, 2 out]
            n1156 = property on="最小允许充电温度" class="DigNum (严格)"("Disabled"=w1858) -> ()  [unwired: 2 in, 2 out]
            n1157 = property on="电流步长" class="DigNum (严格)"("Disabled"=w1858) -> ()  [unwired: 2 in, 2 out]
            n1158 = property on="最大允许单体电压" class="DigNum (严格)"("Disabled"=w1858) -> ()  [unwired: 2 in, 2 out]
            n1159 = property on="最小允许单体电压" class="DigNum (严格)"("Disabled"=w1858) -> ()  [unwired: 2 in, 2 out]
            n1160 = property on="最大允许充电电流" class="DigNum (严格)"("Disabled"=w1858) -> ()  [unwired: 2 in, 2 out]
            n1161 = property on="最小允许充电电流" class="DigNum (严格)"("Disabled"=w1858) -> ()  [unwired: 2 in, 2 out]
          }
          event "1 11": Value Change {
            w1876 = FALSE ("1")
            n1162 = event-data() -> ()  [unwired: 7 out]
            n1163 = local write "主板2"(T8."电池信息" ("主从板")) -> ()
            n1164 = Not(x=w1876) -> (.not. x?=w1875:bool)
            n1165 = local write "1"(w1876) -> ()
            n1166 = local write "1 2"(w1876) -> ()
            n1167 = local write "1 3"(w1876) -> ()
            n1168 = local write "1 4"(w1876) -> ()
            n1169 = local write "1 5"(w1876) -> ()
            n1170 = local write "1 11"(w1875) -> ()
            n1171 = global read "功能码全局.vi" "主板监控2"() -> (w1871:bool[])
            n1172 = Index Array(array=w1871, index=6 ("索引")) -> (element=w1869:bool)
            n1173 = Select(t=0, s=w1869, f=1) -> (s? t:f=w1872:i32)
            n1174 = property on="电池串联" class="DigNum (严格)"("Disabled"=w1872) -> ()  [unwired: 2 in, 2 out]
            n1175 = property on="电池并联" class="DigNum (严格)"("Disabled"=w1872) -> ()  [unwired: 2 in, 2 out]
            n1176 = property on="电池包额定容量" class="DigNum (严格)"("Disabled"=w1872) -> ()  [unwired: 2 in, 2 out]
            n1177 = property on="电池包额定能量(kWh)" class="DigNum (严格)"("Disabled"=w1872) -> ()  [unwired: 2 in, 2 out]
            n1178 = property on="电池包额定总电压" class="DigNum (严格)"("Disabled"=w1872) -> ()  [unwired: 2 in, 2 out]
            n1179 = property on="实际容量" class="DigNum (严格)"("Disabled"=w1872) -> ()  [unwired: 2 in, 2 out]
            n1180 = property on="电池包组号" class="Str"("Disabled"=w1872) -> ()  [unwired: 2 in, 2 out]
            n1181 = property on="电池生产日期" class="Str"("Disabled"=w1872) -> ()  [unwired: 2 in, 2 out]
            n1182 = property on="电池厂家" class="Str"("Disabled"=w1872) -> ()  [unwired: 2 in, 2 out]
            n1183 = property on="电池类型" class="Str"("Disabled"=w1872) -> ()  [unwired: 2 in, 2 out]
            n1184 = property on="累计充电总安时" class="DigNum (严格)"("Disabled"=w1872) -> ()  [unwired: 2 in, 2 out]
            n1185 = property on="累计放电总安时" class="DigNum (严格)"("Disabled"=w1872) -> ()  [unwired: 2 in, 2 out]
            n1186 = property on="电池放空次数" class="DigNum (严格)"("Disabled"=w1872) -> ()  [unwired: 2 in, 2 out]
            n1187 = property on="电池充满次数" class="DigNum (严格)"("Disabled"=w1872) -> ()  [unwired: 2 in, 2 out]
            n1188 = property on="电池充电次数" class="DigNum (严格)"("Disabled"=w1872) -> ()  [unwired: 2 in, 2 out]
            n1189 = property on="电池信息" class="Clust (严格)"("DisabledEnum"=w1872) -> ()  [unwired: 2 in, 2 out]
          }
          event "1 6": Value Change {
            w1887 = FALSE ("1 6")
            n1190 = event-data() -> ()  [unwired: 7 out]
            n1191 = local write "等级 2"(T21."从板信息" ("等级 2")) -> ()
            n1192 = global read "功能码全局.vi" "主板监控2"() -> (w1882:bool[])
            n1193 = Not(x=w1887) -> (.not. x?=w1886:bool)
            n1194 = local write "1 6"(w1886) -> ()
            n1195 = local write "1 7"(w1887) -> ()
            n1196 = local write "1 8"(w1887) -> ()
            n1197 = local write "1 9"(w1887) -> ()
            n1198 = local write "1 10"(w1887) -> ()
            n1199 = Index Array(array=w1882, index=6 ("索引")) -> (element=w1880:bool)
            n1200 = Select(t=0, s=w1880, f=1) -> (s? t:f=w1883:i32)
            n1201 = property on="项目信息 2" class="Tbl (严格)"("Disabled"=w1883) -> ()  [unwired: 2 in, 2 out]
            n1202 = property on="加热控制参数" class="Clust (严格)"("Disabled"=w1883) -> ()  [unwired: 2 in, 2 out]
          }
          event "1 7": Value Change {
            w1898 = FALSE ("1 6")
            n1203 = event-data() -> ()  [unwired: 7 out]
            n1204 = global read "功能码全局.vi" "主板监控2"() -> (w1896:bool[])
            n1205 = Index Array(array=w1896, index=6 ("索引")) -> (element=w1891:bool)
            n1206 = local write "等级 2"(T21."一级故障阀值" ("等级 2")) -> ()
            n1207 = Select(t=0, s=w1891, f=1) -> (s? t:f=w1892:i32)
            n1208 = property on="一级故障 6" class="Clust (严格)"("DisabledEnum"=w1892) -> ()  [unwired: 2 in, 2 out]
            n1209 = Not(x=w1898) -> (.not. x?=w1897:bool)
            n1210 = local write "1 6"(w1898) -> ()
            n1211 = local write "1 7"(w1897) -> ()
            n1212 = local write "1 8"(w1898) -> ()
            n1213 = local write "1 9"(w1898) -> ()
            n1214 = local write "1 10"(w1898) -> ()
          }
          event "1 8": Value Change {
            w1909 = FALSE ("1 6")
            n1215 = event-data() -> ()  [unwired: 7 out]
            n1216 = global read "功能码全局.vi" "主板监控2"() -> (w1907:bool[])
            n1217 = Index Array(array=w1907, index=6 ("索引")) -> (element=w1902:bool)
            n1218 = local write "等级 2"(T21."二级故障阀值" ("等级 2")) -> ()
            n1219 = Select(t=0, s=w1902, f=1) -> (s? t:f=w1903:i32)
            n1220 = Not(x=w1909) -> (.not. x?=w1908:bool)
            n1221 = property on="一级故障 7" class="Clust (严格)"("DisabledEnum"=w1903) -> ()  [unwired: 2 in, 2 out]
            n1222 = local write "1 6"(w1909) -> ()
            n1223 = local write "1 7"(w1909) -> ()
            n1224 = local write "1 8"(w1908) -> ()
            n1225 = local write "1 9"(w1909) -> ()
            n1226 = local write "1 10"(w1909) -> ()
          }
          event "1 9": Value Change {
            w1920 = FALSE ("1 6")
            n1227 = event-data() -> ()  [unwired: 7 out]
            n1228 = global read "功能码全局.vi" "主板监控2"() -> (w1918:bool[])
            n1229 = Index Array(array=w1918, index=6 ("索引")) -> (element=w1913:bool)
            n1230 = Select(t=0, s=w1913, f=1) -> (s? t:f=w1914:i32)
            n1231 = local write "等级 2"(T21."三级故障阀值" ("等级 2")) -> ()
            n1232 = property on="一级故障 8" class="Clust (严格)"("DisabledEnum"=w1914) -> ()  [unwired: 2 in, 2 out]
            n1233 = Not(x=w1920) -> (.not. x?=w1919:bool)
            n1234 = local write "1 6"(w1920) -> ()
            n1235 = local write "1 7"(w1920) -> ()
            n1236 = local write "1 8"(w1920) -> ()
            n1237 = local write "1 9"(w1919) -> ()
            n1238 = local write "1 10"(w1920) -> ()
          }
          event "1 10": Value Change {
            w1931 = FALSE ("1 6")
            n1239 = event-data() -> ()  [unwired: 7 out]
            n1240 = global read "功能码全局.vi" "主板监控2"() -> (w1929:bool[])
            n1241 = Index Array(array=w1929, index=6 ("索引")) -> (element=w1924:bool)
            n1242 = Select(t=0, s=w1924, f=1) -> (s? t:f=w1925:i32)
            n1243 = local write "等级 2"(T21."快换参数" ("等级 2")) -> ()
            n1244 = property on="电池组信息" class="Clust (严格)"("Disabled"=w1925) -> ()  [unwired: 2 in, 2 out]
            n1245 = Not(x=w1931) -> (.not. x?=w1930:bool)
            n1246 = local write "1 6"(w1931) -> ()
            n1247 = local write "1 7"(w1931) -> ()
            n1248 = local write "1 8"(w1931) -> ()
            n1249 = local write "1 9"(w1931) -> ()
            n1250 = local write "1 10"(w1930) -> ()
          }
          event "1 12": Value Change {
            w1936 = FALSE ("1 6")
            n1251 = event-data() -> ()  [unwired: 7 out]
            n1252 = global read "功能码全局.vi" "主板监控2"() -> (w1943:bool[])
            n1253 = Index Array(array=w1943, index=6 ("索引")) -> (element=w1939:bool)
            n1254 = Select(t=0, s=w1939, f=1) -> (s? t:f=w1935:i32)
            n1255 = local write "等级 2"(T14."均衡参数" ("等级 2")) -> ()
            n1256 = property on="均衡参数" class="Clust (严格)"("DisabledEnum"=w1935) -> ()  [unwired: 2 in, 2 out]
            n1257 = Not(x=w1936) -> (.not. x?=w1937:bool)
            n1258 = local write "1 12"(w1937) -> ()
            n1259 = local write "1 6"(w1936) -> ()
            n1260 = local write "1 7"(w1936) -> ()
            n1261 = local write "1 8"(w1936) -> ()
            n1262 = local write "1 9"(w1936) -> ()
            n1263 = local write "1 10"(w1936) -> ()
          }
          event "主板选项": Mouse Down {
            n1264 = event-data() -> ("CtlRef"=w1959:refnum<vi>)  [unwired: 8 out]
            n1265 = global read "功能码全局.vi" "主板监控2"() -> (w1948:bool[])
            n1266 = property class="Tree (严格)"(reference=w1959) -> ("Value"=w1951:string)  [unwired: 1 in, 2 out]
            n1267 = Index Array(array=w1948, index=6 ("索引")) -> (element=w1946:bool)
            n1268 = case shown="\"温度个数\"" w1951 {
              tunnel: [T8."项目信息" ("主从板") T8."项目信息" ("主从板") T8."项目信息" ("主从板") T8."项目信息" ("主从板") T8."项目信息" ("主从板") T8."项目信息" ("主从板") T8."项目信息" ("主从板") T8."项目信息" ("主从板") T8."项目信息" ("主从板") T8."项目信息" ("主从板") T8."项目信息" ("主从板") T8."项目信息" ("主从板") T8."项目信息" ("主从板") T8."项目信息" ("主从板") T8."项目信息" ("主从板") T8."二级故障阀值" ("主从板") T8."三级故障阀值" ("主从板") T8."一级故障阀值" ("主从板") T8."控制参数" ("主从板") T8."控制参数" ("主从板") T8."电池信息" ("主从板") T8."电池信息" ("主从板") T8."电池信息" ("主从板") T8."电池信息" ("主从板") T8."电池信息" ("主从板") T8."项目信息" ("主从板")] -> w1958
              tunnel: [w1969 w1976 w1991 w2008 w2048 w2082 w2129 w2167 w2217 w2252 w2266 w2281 w2296 w2311 w2325 w2338 w2352 w2365 w2379 w2393 w2406 w2420 w2434 w2448 w2462 w2466] -> w1957
              tunnel: [w1970 w1977 w1992 w2009 w2049 w2083 w2130 w2168 w2218 w2253 w2267 w2282 w2297 w2312 w2326 w2338 w2352 w2364 w2379 w2393 w2406 w2420 w2434 w2448 w2462 w2467] -> w1956
              tunnel: [w1970 w1977 w1992 w2009 w2049 w2083 w2130 w2168 w2218 w2253 w2267 w2282 w2297 w2312 w2326 w2339 w2352 w2365 w2379 w2393 w2406 w2420 w2434 w2448 w2462 w2467] -> w1955
              tunnel: [w1970 w1977 w1992 w2009 w2049 w2083 w2130 w2168 w2218 w2253 w2267 w2282 w2297 w2312 w2326 w2338 w2351 w2365 w2379 w2393 w2406 w2420 w2434 w2448 w2462 w2467] -> w1954
              tunnel: [w1970 w1977 w1992 w2009 w2049 w2083 w2130 w2168 w2218 w2253 w2267 w2282 w2297 w2312 w2326 w2338 w2352 w2365 w2378 w2392 w2406 w2420 w2434 w2448 w2462 w2467] -> w1953
              tunnel: [w1970 w1977 w1992 w2009 w2049 w2083 w2130 w2168 w2218 w2253 w2267 w2282 w2297 w2312 w2326 w2338 w2352 w2365 w2379 w2393 w2405 w2419 w2433 w2447 w2461 w2467] -> w1952
              tunnel: [w1962 FALSE w1987 w2000 w2040 w2073 w2120 w2159 w2210 w2247 w2261 w2275 w2289 w2304 w2320 w2334 w2347 w2360 w2374 w2387 w2401 w2414 w2428 w2442 w2456 FALSE] -> w1950
              tunnel: [w1962 TRUE w1984 w1999 w2039 w2074 w2121 w2158 w2209 w2246 w2260 w2274 w2290 w2305 w2319 w2333 w2346 w2359 w2373 w2386 w2400 w2413 w2427 w2441 w2455 FALSE] -> w1949
              tunnel: w1946 -> [w1967 _ w1981 w1996 w2035 w2070 w2117 w2155 w2207 w2243 w2257 w2271 w2286 w2301 w2316 w2330 w2343 w2356 w2370 w2383 w2397 w2410 w2424 w2438 w2452 _]
              frame "项目信息" {
                w1970 = FALSE
                n1269 = Select(t=0, s=w1967, f=1) -> (s? t:f=w1965:i32)
                n1270 = property on="项目信息" class="Tbl (严格)"("Disabled"=w1965) -> ()  [unwired: 2 in, 2 out]
                n1271 = property on="电池实际容量(A)" class="DigNum (严格)"("Disabled"=w1965) -> ()  [unwired: 2 in, 2 out]
                n1272 = property on="使用者" class="DigNum (严格)"("Disabled"=w1965) -> ()  [unwired: 2 in, 2 out]
                n1273 = property on="SOH(%)" class="DigNum (严格)"("Disabled"=w1965) -> ()  [unwired: 2 in, 2 out]
                n1274 = property on="从板个数" class="DigNum (严格)"("NumText.BGColor"=u32 6618880) -> ()  [unwired: 2 in, 2 out]
                n1275 = property on="电池额定容量(A)" class="DigNum (严格)"("Disabled"=w1965) -> ()  [unwired: 2 in, 2 out]
                n1276 = property on="SOC(%)" class="DigNum (严格)"("Disabled"=w1965) -> ()  [unwired: 2 in, 2 out]
                n1277 = property on="项目信息2" class="Clust (严格)"("DisabledEnum"=w1965) -> ()  [unwired: 2 in, 2 out]
                n1278 = property on="系统时钟" class="Str"("Disabled"=w1965) -> ()  [unwired: 2 in, 2 out]
                n1279 = property on="配置文件版本" class="Str"("Disabled"=w1965) -> ()  [unwired: 2 in, 2 out]
                n1280 = property on="车架(牌)号" class="Str"("Disabled"=w1965) -> ()  [unwired: 2 in, 2 out]
                n1281 = property on="产品编号" class="Str"("Disabled"=w1965) -> ()  [unwired: 2 in, 2 out]
                n1282 = local read "项目信息结果"() -> (w1963:bool)
                n1283 = Not(x=w1963) -> (.not. x?=w1962:bool)
                n1284 = Not(x=w1970) -> (.not. x?=w1969:bool)
              }
              frame "校正时钟" {
                w1973 = 2
                w1977 = FALSE
                n1285 = property on="从板个数" class="DigNum (严格)"("NumText.BGColor"=u32 13816530) -> ()  [unwired: 2 in, 2 out]
                n1286 = property on="项目信息" class="Tbl (严格)"("Disabled"=w1973) -> ()  [unwired: 2 in, 2 out]
                n1287 = property on="电池实际容量(A)" class="DigNum (严格)"("Disabled"=w1973) -> ()  [unwired: 2 in, 2 out]
                n1288 = property on="使用者" class="DigNum (严格)"("Disabled"=w1973) -> ()  [unwired: 2 in, 2 out]
                n1289 = property on="SOH(%)" class="DigNum (严格)"("Disabled"=w1973) -> ()  [unwired: 2 in, 2 out]
                n1290 = property on="电池额定容量(A)" class="DigNum (严格)"("Disabled"=w1973) -> ()  [unwired: 2 in, 2 out]
                n1291 = property on="SOC(%)" class="DigNum (严格)"("Disabled"=w1973) -> ()  [unwired: 2 in, 2 out]
                n1292 = property on="系统时钟" class="Str"("Disabled"=w1973) -> ()  [unwired: 2 in, 2 out]
